vi "7067 Relay Module (SubVI).vi"(0 "COM Port":refnum<visa-resource-name>="COM1", 1 "Module Address":i32=1, 2 "Minimum Wait (ms)":u32=100, 3 "Use Master Control?":bool, 5 "Relay Control":T1, 9 "E-STOP (ALL OFF)":bool) -> (14 "Relays Active?":bool, 19 "Error Output":errorcluster)   [LabVIEW 2009]
panel:
  # "7067 - Relay Module (SubVI)\nCreated by Blake Otting 6/13/2007\nUpdated 1/21/2010"
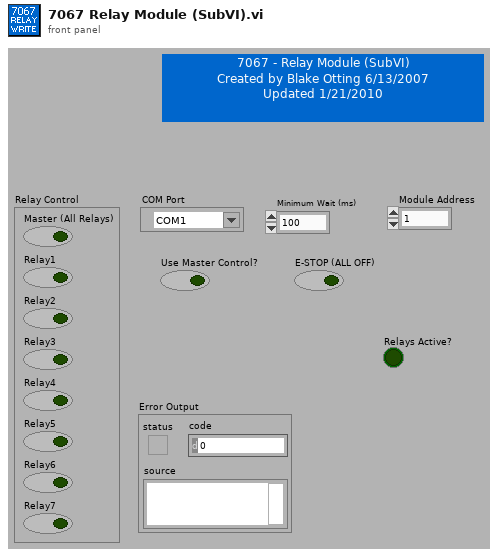
[diagram p1: front panel]
types:
  T1 = cluster{"Master (All Relays)":bool, "Relay1":bool, "Relay2":bool, "Relay3":bool, "Relay4":bool, "Relay5":bool, "Relay6":bool, "Relay7":bool}
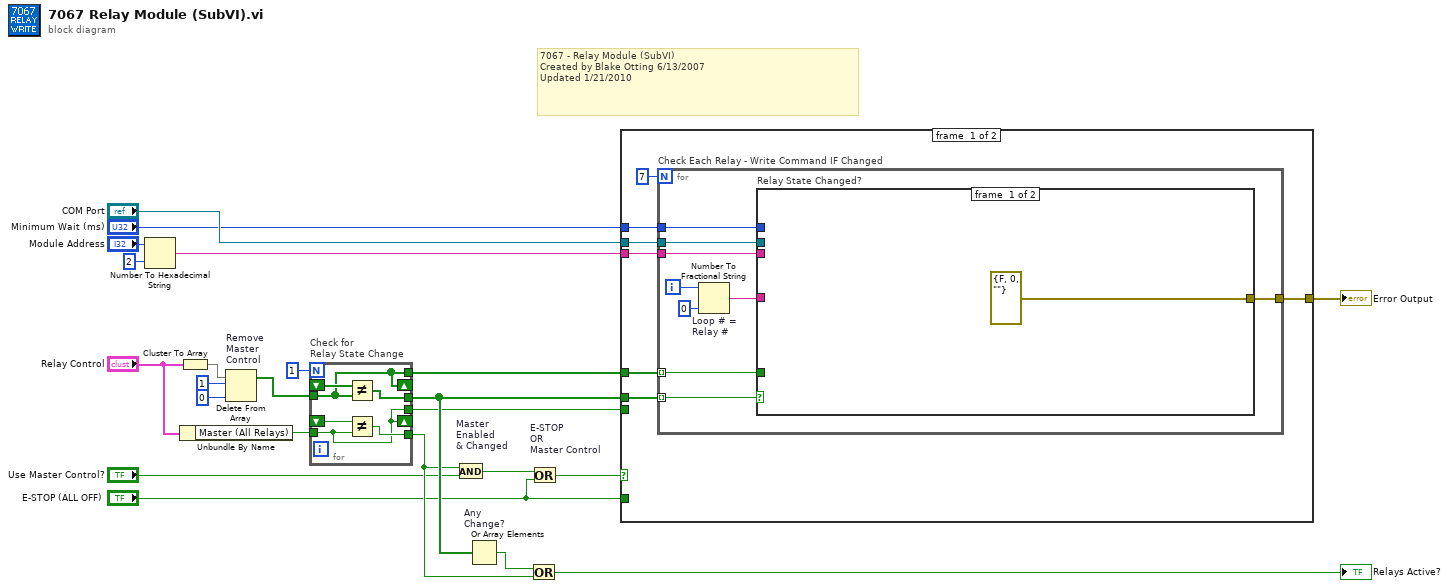
[diagram p0: block diagram]
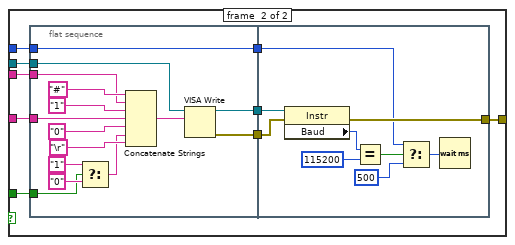
[diagram p2: hidden frame]
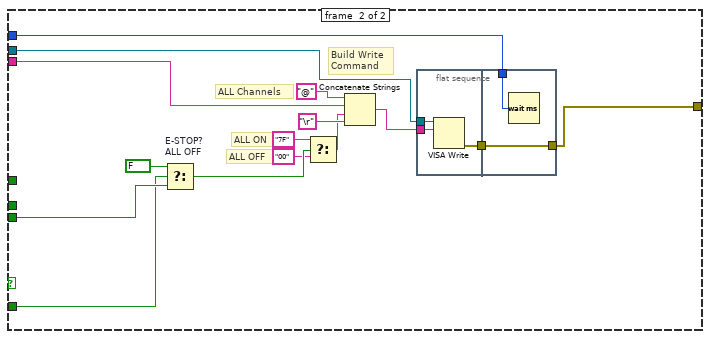
[diagram p3: hidden frame]
diagram:
  # "7067 - Relay Module (SubVI)\nCreated by Blake Otting 6/13/2007\nUpdated 1/21/2010"
  n1 = Number To Hexadecimal String(1:i16 2 ("width (-)"), 2:"Module Address") -> (0:w20:string)
  n2 = Cluster To Array(cluster="Relay Control") -> (array=w16:bool[])
  n3 = Unbundle By Name("Relay Control") -> ("Master (All Relays)"=w13:bool)
  n4 = Delete From Array "Remove\nMaster\nControl"(array=w16, length=1, index=0) -> (array with subset deleted=w6:bool[])  [unwired: 1 out]
  n5 = for "Check for\nRelay State Change" {
    N: 1 -> [_]
    tunnel: w6 -> [w25]
    shift-right: [w25] -> _
    shift-left: _ -> [w29]
    tunnel: [w28] -> w7
    shift-right: [w24] -> _
    shift-left: _ -> [w27]
    tunnel: w13 -> [w24]
    tunnel: [w26] -> w3
    tunnel: [w25] -> w5
    tunnel: [w24] -> w4
    n6 = Not Equal?(x=w29, y=w25) -> (x != y?=w28:bool[])
    n7 = Not Equal?(x=w27, y=w24) -> (x != y?=w26:bool)
  }
  n8 = And "Master\nEnabled\n& Changed"(x=w3, y="Use Master Control?") -> (x .and. y?=w8:bool)
  n9 = Or Array Elements "Any\nChange?"(Boolean array=w7) -> (logical OR=w11:bool)
  n10 = Or(x=w11, y=w3) -> (x .or. y?=→"Relays Active?":bool)
  n11 = Or "E-STOP\nOR\nMaster Control"(x=w8, y="E-STOP (ALL OFF)") -> (x .or. y?=w9:bool)
  n12 = case shown="False" w9 {
    tunnel: w20 -> [w35 w94]
    tunnel: "Minimum Wait (ms)" -> [w34 w80]
    tunnel: "COM Port" -> [w33 w93]
    tunnel: [w32 w92] -> w23
    tunnel: w7 -> [w31 _]
    tunnel: w5 -> [w30 _]
    tunnel: w4 -> [_ w91]
    tunnel: "E-STOP (ALL OFF)" -> [_ w81]
    frame #0 {
      n13 = for "Check Each Relay - Write Command IF Changed" {
        N: 7 -> [_]
        tunnel: w35 -> [w44]
        tunnel: w34 -> [w42]
        tunnel: w33 -> [w41]
        tunnel: [w39] -> w32
        tunnel: w31 -> [w38] mode=indexing
        tunnel: w30 -> [w37] mode=indexing
        i -> [w43]
        n14 = Number To Fractional String "Loop # = \nRelay #"(number=w43, precision (6)=i16 0) -> (F-format string=w45:string)  [unwired: 2 out]
        n15 = case "Relay State Changed?" shown="True" w38 {
          tunnel: w37 -> [_ w55]
          tunnel: w44 -> [_ w54]
          tunnel: w41 -> [_ w53]
          tunnel: w45 -> [_ w50]
          tunnel: w42 -> [_ w49]
          tunnel: [errorcluster {"status"=FALSE, "code"=0, "source"=""} ("error out") w47] -> w39
          frame #0 {
          }
          frame #1 {
            n16 = flat-sequence {
              tunnel: w55 -> [w64]
              tunnel: w54 -> [w63]
              tunnel: w53 -> [w56]
              tunnel: [w60] -> w52
              tunnel: [w59] -> w51
              tunnel: w49 -> [w57]
              tunnel: w50 -> [w58]
              tunnel: [w57] -> w48
              tunnel: w52 -> [w79]
              tunnel: w51 -> [w78]
              tunnel: [w77] -> w47
              tunnel: w48 -> [w72]
              frame #0 {
                n17 = Select(t="1" ("Write Command"), s=w64, f="0" ("Write Command")) -> (s? t:f=w62:string)
                n18 = Concatenate Strings("#" ("Write Command"), w63, "1" ("Write Command"), w58, "0" ("Write Command"), w62, "\r" ("string")) -> (w61:string)
                n19 = VISA Write(VISA resource name=w56, write buffer=w61) -> (VISA resource name out=w60:refnum<visa-resource-name>, error out=w59:errorcluster)  [unwired: 1 in, 1 out]
              }
              frame #1 {
                n20 = property class="Instr"(reference=w79, error in=w78) -> (error out=w77:errorcluster, "Baud"=w76:u32)  [unwired: 1 out]
                n21 = Equal?(x=w76, y=u32 115200) -> (x = y?=w74:bool)
                n22 = Select(t=w72, s=w74, f=u32 500) -> (s? t:f=w71:u32)
                n23 = Wait (ms)(milliseconds to wait=w71) -> ()  [unwired: 1 out]
              }
            }
          }
        }
      }
    }
    frame #1 {
      # "Build Write\nCommand"
      # "ALL Channels"
      # "ALL OFF"
      # "ALL ON"
      n24 = Select "E-STOP?\nALL OFF"(t=FALSE ("E-Stop-ALL OFF"), s=w81, f=w91) -> (s? t:f=w89:bool)
      n25 = Select(t="7F" ("Write Command"), s=w89, f="00" ("Write Command")) -> (s? t:f=w82:string)
      n26 = Concatenate Strings("@" ("string"), w94, w82, "\r" ("string")) -> (w87:string)
      n27 = flat-sequence {
        tunnel: w87 -> [w97]
        tunnel: w93 -> [w96]
        tunnel: [w95] -> w90
        tunnel: [w99] -> w92
        tunnel: w90 -> [w99]
        tunnel: w80 -> [w98]
        frame #0 {
          n28 = VISA Write(VISA resource name=w96, write buffer=w97) -> (error out=w95:errorcluster)  [unwired: 1 in, 2 out]
        }
        frame #1 {
          n29 = Wait (ms)(milliseconds to wait=w98) -> ()  [unwired: 1 out]
        }
      }
    }
  }
  "Error Output" <- w23
